vi "外观.vi"(0 "Data In":T7 caption="数据输入", 2 "Display State In":T4={"完成"=FALSE, "功能选择"=enum."扫描", "数据"=[], "历史数据"=[], "曲线设置"={"X"=enum."设置电压", "Y1"=enum."读取电流", "Y2"=enum."无", "Y3"=enum."无"}, "突变电压"=refnum, "保留数量"=0, "属性"=variant} caption="显示状态输入", 3 "Container State":T6 caption="容器状态") -> (6 "Data Out":T7 caption="数据输出", 7 "Display State Out":T4={"完成"=FALSE, "功能选择"=enum."扫描", "数据"=[], "历史数据"=[], "曲线设置"={"X"=enum."设置电压", "Y1"=enum."读取电流", "Y2"=enum."无", "Y3"=enum."无"}, "突变电压"=refnum, "保留数量"=0, "属性"=variant} caption="显示状态输出", 8 "Action":T3 caption="动作")   [LabVIEW 2020, in "数据显示.xctl"]
uses:
  <vilib>/_xctls/Container State.ctl
  <vilib>/_xctls/Action.ctl
  <vilib>/Utility/miscctls.llb/LVAnnotationListTypeDef.ctl
  <vilib>/_xctls/XControlSupport.lvlib
panel:
  in  "监测曲线":i32(ring)
  in  "保留数量":i32=1 min=1 max=20 step=1
  in  "曲线设置":T1={"X"=enum."设置电压", "Y1"=enum."读取电流", "Y2"=enum."无", "Y3"=enum."无"}
  in  "映射方式":T2
  out "刷新":bool
  out "XY图":cluster{dbl[], dbl[]}[](graph)
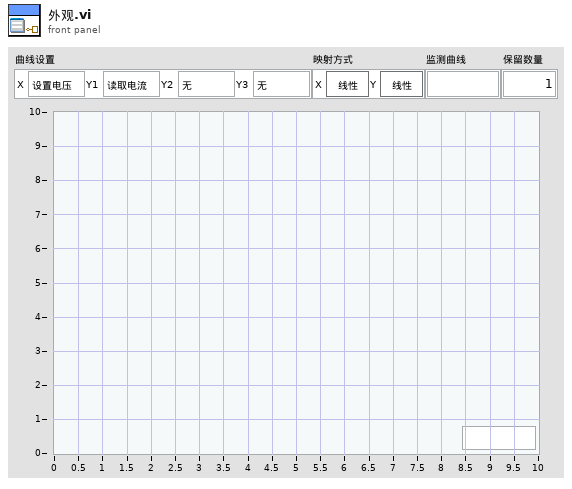
[diagram p1: front panel]
types:
  T1 = typedef "数据显示.xctl/曲线设置.ctl" = cluster{"X":enum16{"时间", "设置电压", "读取电流", "读取电压"}, "Y1":enum16{"时间", "设置电压", "读取电流", "读取电压"}, "Y2":enum16{"时间", "设置电压", "读取电流", "读取电压", "无"}, "Y3":enum16{"时间", "设置电压", "读取电流", "读取电压", "无"}}
  T2 = typedef "数据显示.xctl/映射方式.ctl" = cluster{"X":bool, "Y":bool}
  T3 = typedef "XControlSupport.lvlib/Action.ctl" = cluster{"Data Changed?":bool, "State Changed?":bool, "Action Name":string}
  T4 = typedef "数据显示.xctl/状态.ctl" = cluster{"完成":bool, "功能选择":enum16{"扫描", "循环扫描", "保持时间", "脉冲", "高速脉冲", "任意波形"}, "数据":dbl[][], "历史数据":T5[], "曲线设置":T1, "突变电压":refnum<user-event>, "保留数量":i32, "属性":variant}
  T5 = typedef "数据显示.xctl/波形数据定义.ctl" = cluster{"波形":dbl[][], "属性":variant}
  T6 = typedef "XControlSupport.lvlib/Container State.ctl" = cluster{"Indicator?":bool, "Run Mode?":bool, " Refnum":refnum<vi>}
  T7 = typedef "数据显示.xctl/数据.ctl" = dbl[][]
  T8 = cluster{"Name":string, "Color":u32, "Style":u8, "Point Style":u8, "Name Visible":bool, "Allow Drag":bool, "Annotation Mode":u32, "Plot":i32, "Index":i32, "Position":cluster{"X":dbl, "Y":dbl}, "X Scale":u32, "Y Scale":u32, "Show Arrow":bool, "Lock Name":bool, "Plot Area":i32, "Label Offset":cluster{"X":dbl, "Y":dbl}}
  T9 = typedef "LVAnnotationListTypeDef.ctl" = cluster{"Name":string, "Color":u32, "Style":u8, "Point Style":u8, "Name Visible":bool, "Allow Drag":bool, "Annotation Mode":u32, "Plot":i32, "Index":i32, "Position":cluster{"X":dbl, "Y":dbl}, "X Scale":u32, "Y Scale":u32, "Show Arrow":bool, "Lock Name":bool, "Plot Area":i32, "Label Offset":cluster{"X":dbl, "Y":dbl}}[]
  T10 = enum8{"Enabled", "Disabled", "Disabled and Grayed Out"}
  T11 = enum16{"扫描", "循环扫描", "保持时间", "脉冲", "高速脉冲", "任意波形"}
  T12 = typedef "LVRectTypeDef.ctl" = cluster{"Left":i16, "Top":i16, "Right":i16, "Bottom":i16}
  T13 = cluster{"Name":string, "Color":u32, "Style":u8, "Point Style":u8, "Name Visible":bool, "Allow Drag":bool, "Annotation Mode":u32, "Plot":i32, "Index":i32, "Position":cluster{"X":dbl, "Y":dbl}, "X Scale":u32, "Y Scale":u32, "Show Arrow":bool, "Lock Name":bool, "Plot Area":i32, "Label Offset":cluster{"X":dbl, "Y":dbl}}[]
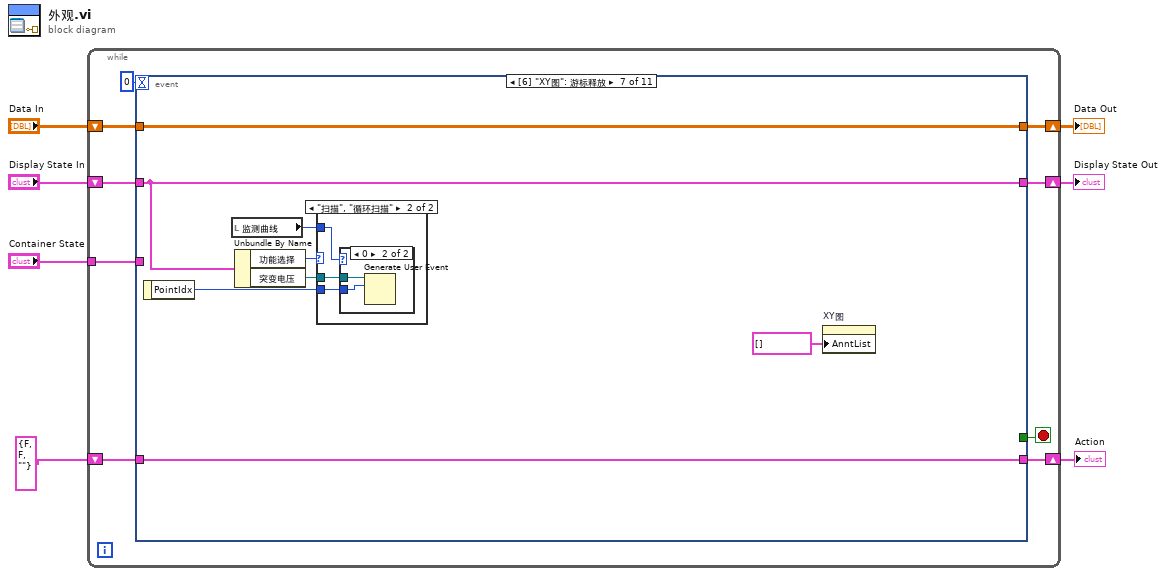
[diagram p0: block diagram]
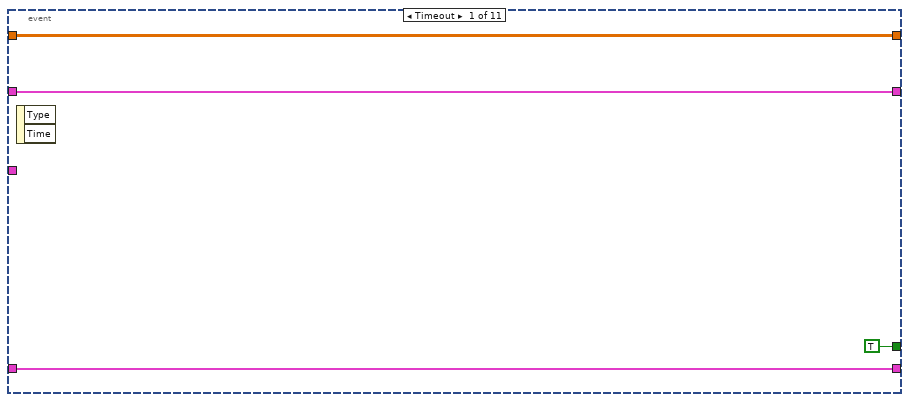
[diagram p2: hidden frame]
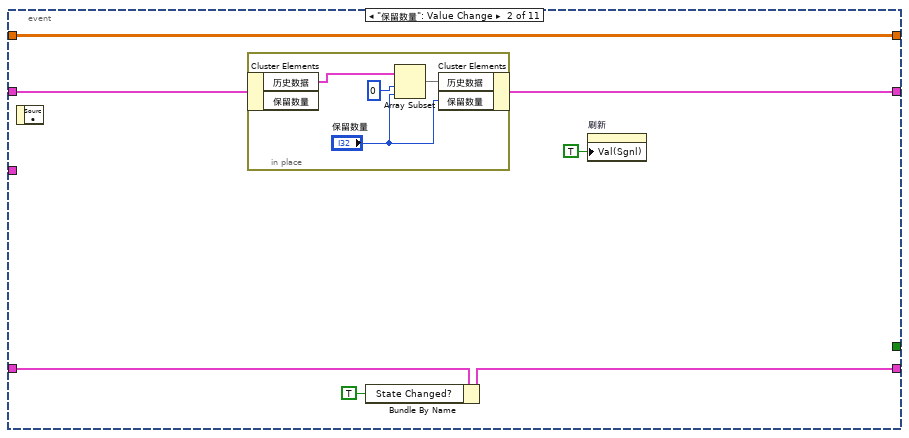
[diagram p3: hidden frame]
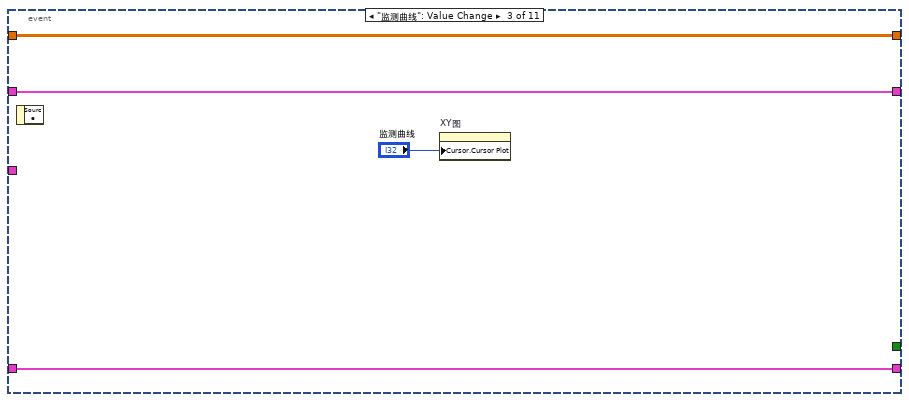
[diagram p4: hidden frame]
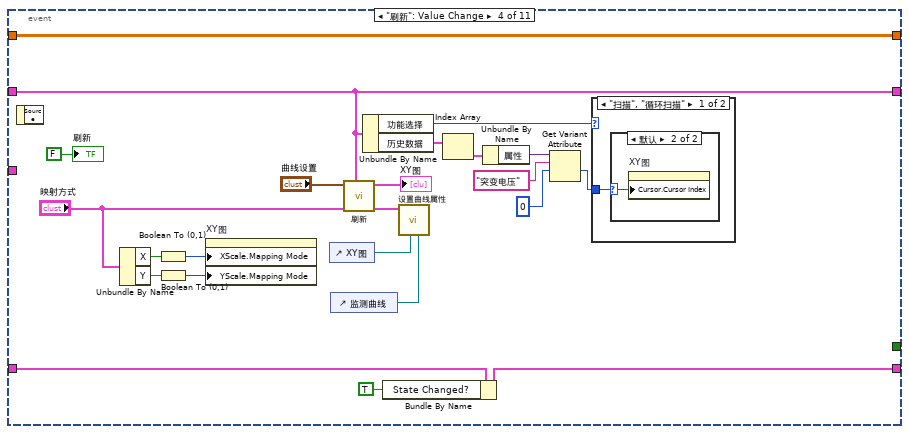
[diagram p5: hidden frame]
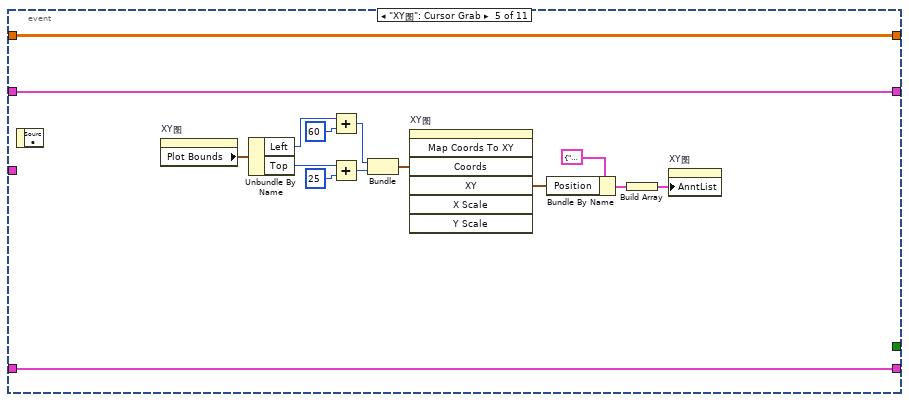
[diagram p8: hidden frame]
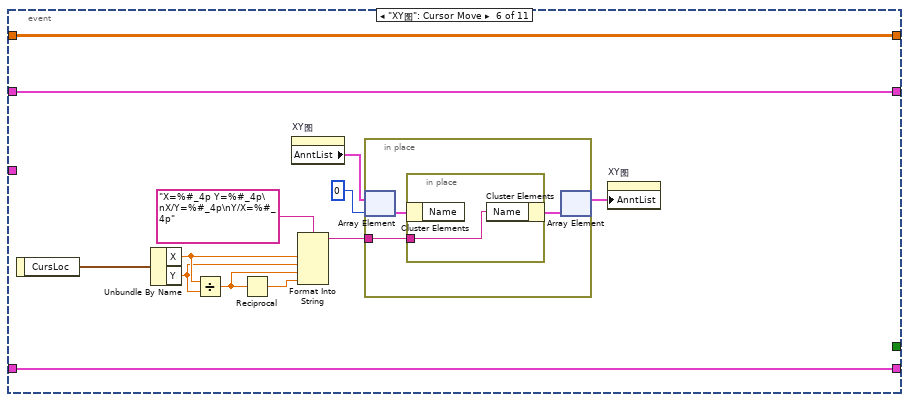
[diagram p9: hidden frame]
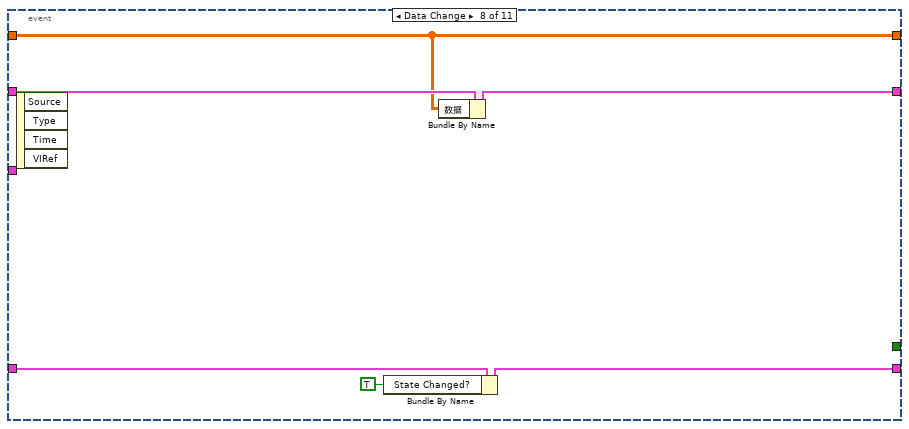
[diagram p12: hidden frame]
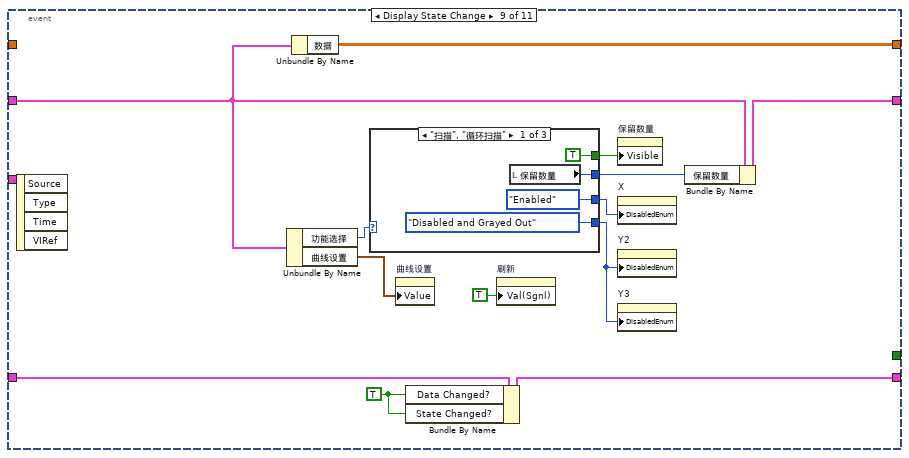
[diagram p13: hidden frame]
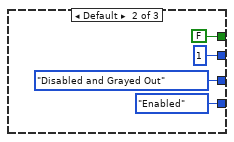
[diagram p14: hidden frame]
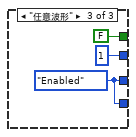
[diagram p15: hidden frame]
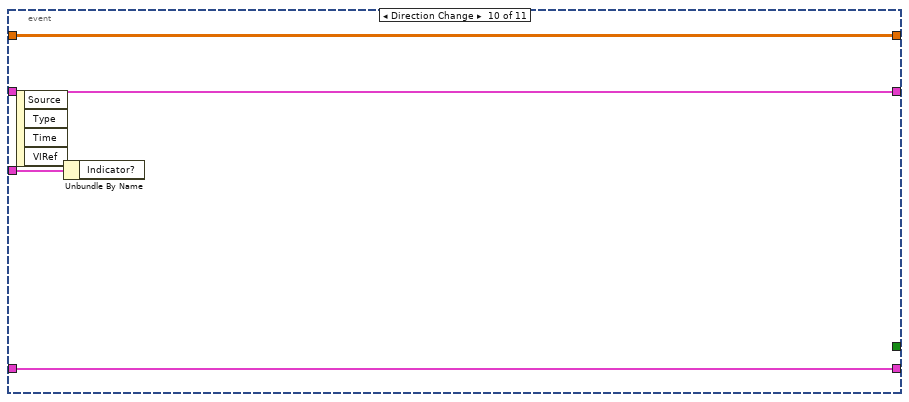
[diagram p16: hidden frame]
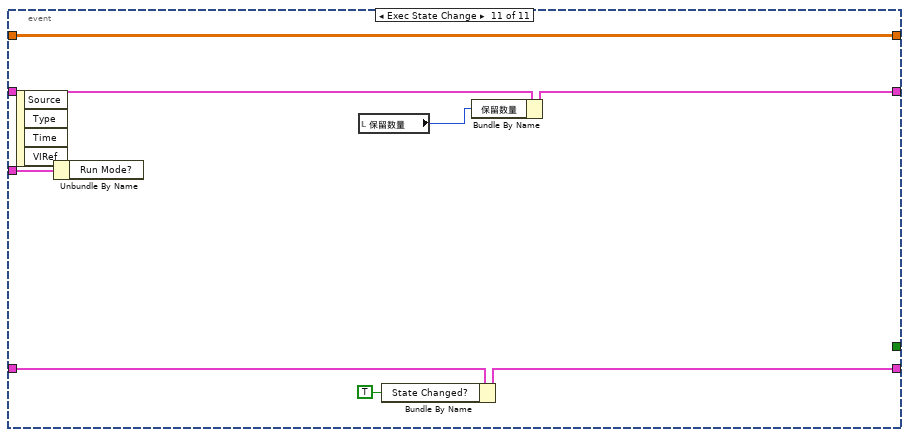
[diagram p17: hidden frame]
diagram:
  n1 = while {
    shift-right: [w15] -> w4
    shift-left: "Display State In" -> [w16]
    tunnel: "Container State" -> [w12]
    shift-right: [w10] -> w7
    shift-left: "Data In" -> [w11]
    shift-right: [w8] -> w2
    shift-left: T3 {"Data Changed?"=FALSE, "State Changed?"=FALSE, "Action Name"=""} ("Action") -> [w9]
    stop <- w14 stop-if-true
    n2 = event shown="[6] \"XY图\": 游标释放" {
      selector: _ -> [_ _ _ _ _ _ _ _ _ _ _]
      dyn-events: _ -> [_ _ _ _ _ _ _ _ _ _ _]
      timeout: 0 -> [_ _ _ _ _ _ _ _ _ _ _]
      tunnel: w16 -> [w18 w27 w35 w43 w75 w88 w97 w111 w120 w138 w146]
      tunnel: [w18 w24 w35 w43 w75 w88 w97 w109 w115 w138 w143] -> w15
      tunnel: [TRUE _ _ _ _ _ _ _ _ _ _] -> w14
      tunnel: w12 -> [_ _ _ _ _ _ _ _ _ w139 w147]
      tunnel: w11 -> [w17 w26 w34 w58 w74 w87 w100 w108 _ w137 w145]
      tunnel: [w17 w26 w34 w58 w74 w87 w100 w108 w123 w137 w145] -> w10
      tunnel: [w19 w23 w33 w56 w73 w86 w99 w107 w122 w136 w142] -> w8
      tunnel: w9 -> [w19 w25 w33 w57 w73 w86 w99 w110 w124 w136 w144]
      event Timeout {
        n3 = event-data() -> ()  [unwired: 1 in, 2 out]
      }
      event "保留数量": Value Change {
        n4 = event-data() -> ()  [unwired: 1 in, 1 out]
        n5 = in-place {
          n6 = in-place-cluster #1(w27) -> ("历史数据"=w31:T5[])  [unwired: 1 out]
          n7 = Array Subset(array=w31, index=0 ("索引"), length="保留数量") -> (w30:T5[])
          n8 = in-place-cluster #1("历史数据"=w30, "保留数量"="保留数量") -> (w24:T4)
        }
        n9 = Bundle By Name(cluster=w25, "State Changed?"=TRUE) -> (w23:T3)
        n10 = property on="刷新" class="Bool (严格)"("Val(Sgnl)"=TRUE ("值(信号)")) -> ()  [unwired: 2 in, 2 out]
      }
      event "监测曲线": Value Change {
        n11 = event-data() -> ()  [unwired: 1 in, 1 out]
        n12 = property on="XY图" class="XYGraph (严格)"("Cursor.Cursor Plot"="监测曲线") -> ()  [unwired: 2 in, 2 out]
      }
      event "刷新": Value Change {
        n13 = event-data() -> ()  [unwired: 1 in, 1 out]
        n14 = Unbundle By Name("映射方式") -> ("X"=w52:bool, "Y"=w51:bool)
        n15 = Boolean To (0,1)(Boolean=w52) -> (0, 1=w50:i16)
        n16 = Boolean To (0,1)(Boolean=w51) -> (0, 1=w49:i16)
        n17 = property on="XY图" class="XYGraph (严格)"("XScale.Mapping Mode"=w50, "YScale.Mapping Mode"=w49) -> ()  [unwired: 2 in, 2 out]
        n18 = control-ref of="XY图"() -> (w47:refnum<vi>)
        n19 = control-ref of="监测曲线"() -> (w48:refnum<vi>)
        n20 = call "刷新.vi"("Display State In"=w43, "映射方式"="映射方式", "曲线设置"="曲线设置") -> ("曲线属性"=w44:cluster{"曲线名":string, "曲线颜色":u32, "线条宽度":u8}[], "XY图"=→"XY图":cluster{"数据":dbl[], "数据":dbl[]}[])  [unwired: 7 in]
        n21 = Unbundle By Name(w43) -> ("功能选择"=w36:T11, "历史数据"=w42:T5[])
        n22 = Bundle By Name(cluster=w57, "State Changed?"=TRUE) -> (w56:T3)
        n23 = call "设置曲线属性.vi"("监测曲线"=w48, "XY图输入"=w47, "曲线属性"=w44) -> ()  [unwired: 9 in]
        n24 = Index Array(array=w42) -> (element=w41:T5)  [unwired: 1 in]
        n25 = Unbundle By Name(w41) -> ("属性"=w40:variant)
        n26 = Get Variant Attribute(Variant=w40, name="突变电压" ("名称"), default value (empty Variant)=0 ("游标.游标索引")) -> (value=w37:i32)  [unwired: 1 in, 3 out]
        n27 = case shown="\"扫描\", \"循环扫描\"" w36 {
          tunnel: w37 -> [w59 _]
          frame "扫描", "循环扫描" {
            n28 = case shown="默认" w59 {
              selector: w59 -> [_ w60]
              frame 0 {
              }
              frame Default {
                n29 = property on="XY图" class="XYGraph (严格)"("Cursor.Cursor Index"=w60) -> ()  [unwired: 2 in, 2 out]
              }
            }
          }
          frame Default {
          }
        }
        "刷新" <- FALSE ("刷新")
      }
      event "XY图": Cursor Grab {
        n30 = event-data() -> ()  [unwired: 1 in, 1 out]
        n31 = property on="XY图" class="XYGraph (严格)"() -> ("Plot Bounds"=w72:T12)  [unwired: 2 in, 2 out]
        n32 = Unbundle By Name(w72) -> ("Left"=w68:i16, "Top"=w71:i16)
        n33 = Add(x=w68, y=i16 60) -> (x+y=w66:i16)
        n34 = Add(x=w71, y=i16 25) -> (x+y=w65:i16)
        n35 = Bundle(w66, w65) -> (w64:cluster{i16, i16})  [unwired: 1 in]
        n36 = invoke on="XY图" class="XYGraph (严格)" method="Map Coords To XY"("Coords"=w64) -> ("XY"=w67:cluster{"X":dbl, "Y":dbl})  [unwired: 6 in, 6 out]
        n37 = Bundle By Name(cluster=T8 {"Name"="", "Color"=0, "Style"=0, "Point Style"=0, "Name Visible"=TRUE, "Allow Drag"=FALSE, "Annotation Mode"=0, "Plot"=-1, "Index"=0, "Position"={"X"=0.0, "Y"=0.0}, "X Scale"=0, "Y Scale"=0, "Show Arrow"=FALSE, "Lock Name"=FALSE, "Plot Area"=0, "Label Offset"={"X"=0.0, "Y"=0.0}} ("元素"), "Position"=w67) -> (w63:T8)
        n38 = Build Array(w63) -> (w62:T13)
        n39 = property on="XY图" class="XYGraph (严格)"("AnntList"=w62) -> ()  [unwired: 2 in, 2 out]
      }
      event "XY图": Cursor Move {
        n40 = event-data() -> ("CursLoc"=w76:cluster{"X":dbl, "Y":dbl})  [unwired: 1 in]
        n41 = Unbundle By Name(w76) -> ("X"=w78:dbl, "Y"=w77:dbl)
        n42 = Divide(x=w78, y=w77) -> (x/y=w85:dbl)
        n43 = Reciprocal(x=w85) -> (1/x=w84:dbl)
        n44 = property on="XY图" class="XYGraph (严格)"() -> ("AnntList"=w82:T9)  [unwired: 2 in, 2 out]
        n45 = Format Into String(format string="X=%#_4p Y=%#_4p\nX/Y=%#_4p\nY/X=%#_4p" ("格式字符串"), w78, w77, w85, w84) -> (resulting string=w80:string)  [unwired: 2 in, 1 out]
        n46 = in-place {
          in-place-border: w80 -> [w89]
          n47 = in-place-array #2(w82, 0) -> (w91:T8)
          n48 = in-place {
            in-place-border: w89 -> [w92]
            n49 = in-place-cluster #3(w91) -> ()  [unwired: 1 out]
            n50 = in-place-cluster #3("Name"=w92) -> (w90:T8)
          }
          n51 = in-place-array #2(w90) -> (w81:T9)  [unwired: 1 out]
        }
        n52 = property on="XY图" class="XYGraph (严格)"("AnntList"=w81) -> ()  [unwired: 2 in, 2 out]
      }
      event "XY图": Cursor Release {
        n53 = event-data() -> ("PointIdx"=w95:i32)  [unwired: 1 in]
        n54 = local read "监测曲线"() -> (w93:i32)
        n55 = Unbundle By Name(w97) -> ("功能选择"=w94:T11, "突变电压"=w96:refnum<user-event>)
        n56 = case shown="\"扫描\", \"循环扫描\"" w94 {
          tunnel: w96 -> [_ w103]
          tunnel: w95 -> [_ w102]
          tunnel: w93 -> [_ w101]
          frame Default {
          }
          frame "扫描", "循环扫描" {
            n57 = case shown="0" w101 {
              tunnel: w103 -> [_ w105]
              tunnel: w102 -> [_ w104]
              frame Default {
              }
              frame 0 {
                n58 = Generate User Event(user event=w105, event data cluster=w104) -> ()  [unwired: 2 in, 2 out]
              }
            }
          }
        }
        n59 = property on="XY图" class="XYGraph (严格)"("AnntList"=T9 [] ("注释列表")) -> ()  [unwired: 2 in, 2 out]
      }
      event Data Change {
        n60 = event-data() -> ()  [unwired: 1 in, 4 out]
        n61 = Bundle By Name(cluster=w110, "State Changed?"=TRUE ("Data Changed?")) -> (w107:T3)
        n62 = Bundle By Name(cluster=w111, "数据"=w108) -> (w109:T4)
      }
      event Display State Change {
        w113 = TRUE ("Data Changed?")
        n63 = event-data() -> ()  [unwired: 1 in, 4 out]
        n64 = Unbundle By Name(w120) -> ("功能选择"=w119:T11, "曲线设置"=w117:T1)
        n65 = Unbundle By Name(w120) -> ("数据"=w123:dbl[][])
        n66 = case shown="\"扫描\", \"循环扫描\"" w119 {
          tunnel: [T10."Disabled and Grayed Out" ("禁用") T10."Enabled" ("禁用") w133] -> w116
          tunnel: [w127 1 ("保留数量") 1 ("保留数量")] -> w114
          tunnel: [TRUE ("可见") FALSE ("可见") FALSE ("可见")] -> w118
          tunnel: [T10."Enabled" ("禁用") T10."Disabled and Grayed Out" ("禁用") w133] -> w112
          frame "扫描", "循环扫描" {
            n67 = local read "保留数量"() -> (w127:i32)
          }
          frame Default {
          }
          frame "任意波形" {
            w133 = T10."Enabled" ("禁用")
          }
        }
        n68 = property on="曲线设置" class="Clust (严格)"("Value"=w117) -> ()  [unwired: 2 in, 2 out]
        n69 = Bundle By Name(cluster=w124, "Data Changed?"=w113, "State Changed?"=w113) -> (w122:T3)
        n70 = property on="刷新" class="Bool (严格)"("Val(Sgnl)"=TRUE ("值(信号)")) -> ()  [unwired: 2 in, 2 out]
        n71 = property on="保留数量" class="DigNum (严格)"("Visible"=w118) -> ()  [unwired: 2 in, 2 out]
        n72 = property on="X" class="Enum (严格)"("DisabledEnum"=w112) -> ()  [unwired: 2 in, 2 out]
        n73 = property on="Y2" class="Enum (严格)"("DisabledEnum"=w116) -> ()  [unwired: 2 in, 2 out]
        n74 = property on="Y3" class="Enum (严格)"("DisabledEnum"=w116) -> ()  [unwired: 2 in, 2 out]
        n75 = Bundle By Name(cluster=w120, "保留数量"=w114) -> (w115:T4)
      }
      event Direction Change {
        n76 = event-data() -> ()  [unwired: 1 in, 4 out]
        n77 = Unbundle By Name(w139) -> ()  [unwired: 1 out]
      }
      event Exec State Change {
        n78 = event-data() -> ()  [unwired: 1 in, 4 out]
        n79 = Unbundle By Name(w147) -> ()  [unwired: 1 out]
        n80 = local read "保留数量"() -> (w140:i32)
        n81 = Bundle By Name(cluster=w144, "State Changed?"=TRUE) -> (w142:T3)
        n82 = Bundle By Name(cluster=w146, "保留数量"=w140) -> (w143:T4)
      }
    }
  }
  "Display State Out" <- w4
  "Data Out" <- w7
  "Action" <- w2
